vi "test Add Find Remove Analog Replay No VOverride.vi"(8 "error in (no error)":errorcluster, 11 "TestCase in":refnum<class "Scripting API Test Case.lvclass">) -> (0 "error out":errorcluster, 3 "TestCase out":refnum<class "Scripting API Test Case.lvclass">)   [LabVIEW 2019, in "Scripting API Test Case.lvclass"]
uses:
  Scripting API Test Case.lvclass
  <vilib>/addons/_JKI Toolkits/VI Tester/TestCase.llb/TestCase.lvclass
  <vilib>/NI/VeriStand Custom Device Testing Tools/VeriStandTestUtilities/VeriStandTestUtilities.lvlib
  Scripting API/Engine Simulation Toolkit Scripting API.lvlib
  Scripting API/Custom Device/Engine Simulation Toolkit Custom Device Settings.ctl
  <userlib>/_OpenG.lib/file/file.llb/Append Path to Root if Relative - Scalar__ogtk.vi
  Scripting API/Bitfile/Bitfile.ctl
  Scripting API/Analog Replay/Analog Replay Settings.ctl
  System Explorer/FPGA Mem Size.ctl
  System Explorer/Engine Simulation Toolkit System Explorer.lvlib
  System Explorer/Position Reference.ctl
  System Explorer/Data Replay Data Selection Method.ctl
  Scripting API/Analog Replay/Analog Replay Data Options.ctl
  C:/Program Files (x86)/National Instruments/LabVIEW 2019/vi.lib/addons/_JKI Toolkits/VI Tester/TestCase.llb/TestCase.lvclass
panel:
  in  "Save?":bool
  out "Output Filename":string
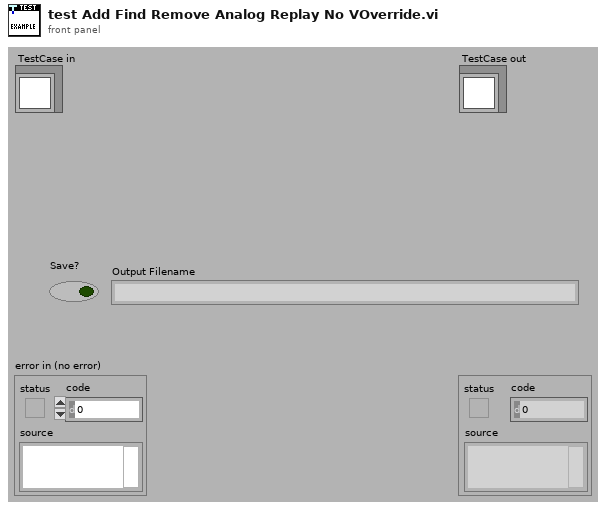
[diagram p1: front panel]
types:
  T1 = typedef "Engine Simulation Toolkit Scripting API.lvlib/Analog Replay Data Options.ctl" = cluster{"Selected File":path, "Group":string, "Channel":string, "DataPlugin":string, "ReverseData":bool, "FPGA memory size":T2, "CycleAngle?":T3, "Data Selection Method":T4, "File start offset":i32, "Samples":i32, "Missing teeth location (degrees)":dbl}
  T2 = typedef "Engine Simulation Toolkit System Explorer.lvlib/FPGA Mem Size.ctl" = enum16{"65,536", "32,768", "16,384", "8,192", "4,096", "2,048", "1,024"}
  T3 = typedef "Engine Simulation Toolkit System Explorer.lvlib/Position Reference.ctl" = enum16{"Crank angle", "Cycle angle"}
  T4 = typedef "Engine Simulation Toolkit System Explorer.lvlib/Data Replay Data Selection Method.ctl" = enum32{"Manual", "AutoVRCrank"}
  T5 = typedef "Engine Simulation Toolkit Scripting API.lvlib/Bitfile.ctl" = cluster{"RIO Device Address":string, "Bitfile Path":path}
  T6 = typedef "Engine Simulation Toolkit Scripting API.lvlib/Engine Simulation Toolkit Custom Device Settings.ctl" = cluster{"Name":string, "Execution priority":enum16{"Low", "Medium", "High"}, "Rate decimation":i32, "CPU":i32}
  T7 = typedef "Engine Simulation Toolkit Scripting API.lvlib/Analog Replay Settings.ctl" = cluster{"Name":string, "RIO Device Address":string, "DAC bipolar range (V)":dbl, "Voltage below min speed":dbl, "Min speed (RPM)":dbl, "Voltage at min speed":dbl, "Max speed (RPM)":dbl, "Voltage at max speed":dbl, "ReverseNegate":bool, "VOverride":bool}
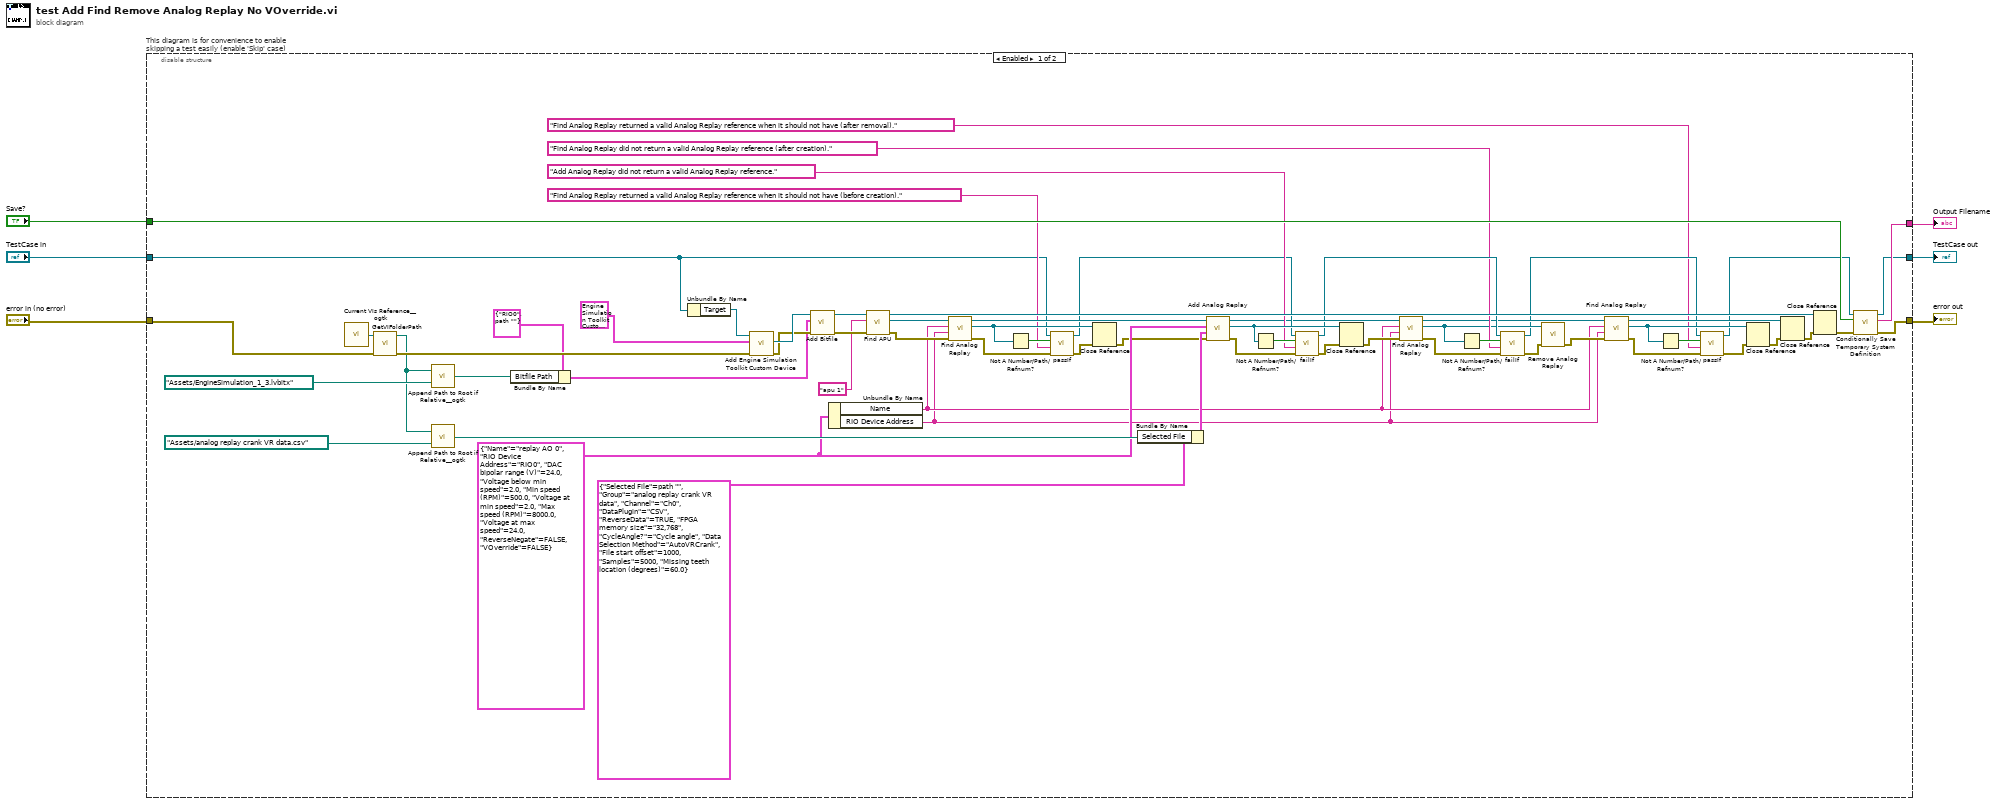
[diagram p0: block diagram]
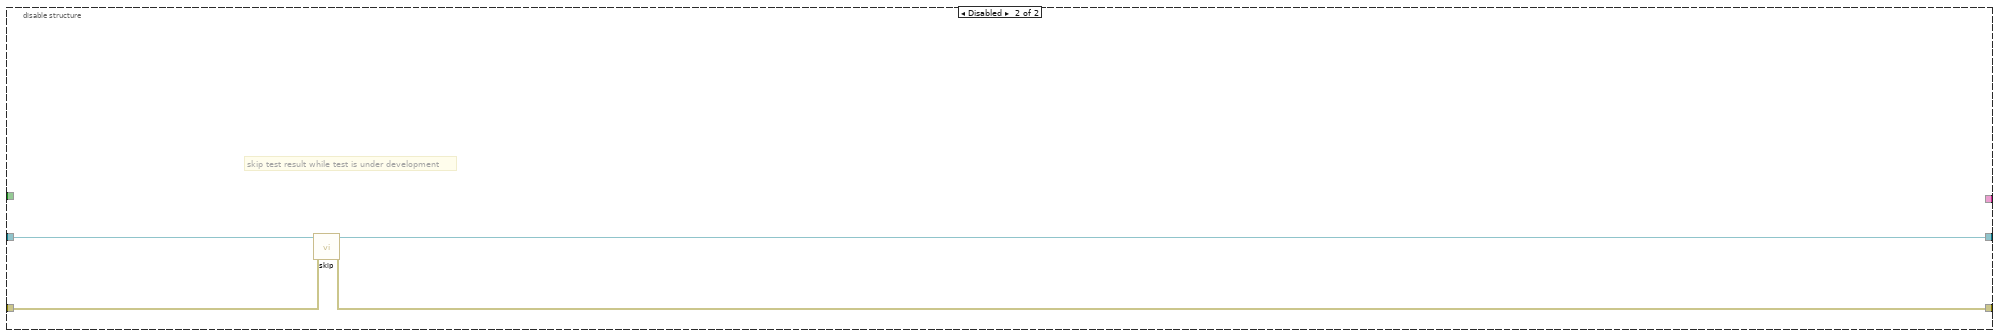
[diagram p2: hidden frame]
diagram:
  n1 = disable-structure "This diagram is for convenience to enable skipping a test easily (enable 'Skip' case)" shown="Enabled" {
    disable-tunnel: "TestCase in" -> [w8 w74]
    disable-tunnel: [w9 w72] -> w3
    disable-tunnel: [w66 w73] -> w5
    disable-tunnel: "error in (no error)" -> [w69 w71]
    disable-tunnel: [w65 _] -> w2
    disable-tunnel: "Save?" -> [w64 _]
    frame Enabled {
      w41 = T7 {"Name"="replay AO 0", "RIO Device Address"="RIO0", "DAC bipolar range (V)"=24.0, "Voltage below min speed"=2.0, "Min speed (RPM)"=500.0, "Voltage at min speed"=2.0, "Max speed (RPM)"=8000.0, "Voltage at max speed"=24.0, "ReverseNegate"=FALSE, "VOverride"=FALSE} ("Analog Replay Settings")
      n2 = call <userlib>:"Current VIs Reference__ogtk.vi"() -> ("Current VI's reference"=w70:refnum<vi>)  [unwired: 5 in]
      n3 = call <vilib>:"GetVIFolderPath.vi"("error in (no error)"=w69, "VI Reference in"=w70) -> ("error out"=w68:errorcluster, "VI Folder Path out"=w49:path)  [unwired: 8 in]
      n4 = call-poly <userlib>:"Append Path to Root if Relative__ogtk.vi"("Absolute or Relative Path"=path "Assets/EngineSimulation_1_3.lvbitx", "Root Path"=w49) -> ("Absolute or Appended Path"=w57:path)
      n5 = call-poly <userlib>:"Append Path to Root if Relative__ogtk.vi"("Absolute or Relative Path"=path "Assets/analog replay crank VR data.csv", "Root Path"=w49) -> ("Absolute or Appended Path"=w48:path)
      n6 = Bundle By Name(cluster=T5 {"RIO Device Address"="RIO0", "Bitfile Path"=path ""} ("Engine Simulation Toolkit Bitfile"), "Bitfile Path"=w57) -> (w58:T5)
      n7 = Unbundle By Name(w8) -> ("Target"=w7:refnum<k24>)
      n8 = call "Add Engine Simulation Toolkit Custom Device.vi"("error in (no error)"=w68, "Settings"=T6 {"Name"="Engine Simulation Toolkit Custom Device", "Execution priority"=enum."Medium", "Rate decimation"=1, "CPU"=-2} ("Engine Simulation Toolkit Custom Device Settings"), "Target in"=w7) -> ("error out"=w61:errorcluster, "EST Custom Device"=w63:refnum<k24>)  [unwired: 6 in, 1 out]
      n9 = call "Add Bitfile.vi"("error in (no error)"=w61, "Engine Simulation Toolkit Bitfile"=w58, "EST Custom Device in"=w63) -> ("error out"=w55:errorcluster, "EST Custom Device out"=w56:refnum<k24>)  [unwired: 7 in]
      n10 = Unbundle By Name(w41) -> ("Name"=w20:string, "RIO Device Address"=w19:string)
      n11 = call "Find APU.vi"("error in (no error)"=w55, "Name"="apu 1", "EST Custom Device in"=w56) -> ("error out"=w38:errorcluster, "APU"=w40:refnum<k24>, "EST Custom Device out"=w54:refnum<k24>)  [unwired: 6 in]
      n12 = call "Find Analog Replay.vi"("error in (no error)"=w38, "RIO Device Address"=w19, "Name"=w20, "APU in"=w40) -> ("error out"=w34:errorcluster, "Analog Replay"=w36:refnum<k24>, "APU out"=w39:refnum<k24>)  [unwired: 5 in]
      n13 = Not A Number/Path/Refnum?(number/path/refnum=w36) -> (NaN/Path/Refnum?=w37:bool)
      n14 = call-dynamic "passIf.vi"("error in (no error)"=w34, "message (\"\")"="Find Analog Replay returned a valid Analog Replay reference when it should not have (before creation)." ("message (\"\")"), "pass"=w37, "TestCase in"=w8) -> ("error out"=w35:errorcluster, "TestCase out"=w33:refnum<class "Scripting API Test Case.lvclass">)  [unwired: 6 in]
      n15 = Close Reference(reference=w36, error in (no error)=w35) -> (error out=w31:errorcluster)
      n16 = Bundle By Name(cluster=T1 {"Selected File"=path "", "Group"="analog replay crank VR data", "Channel"="Ch0", "DataPlugin"="CSV", "ReverseData"=TRUE, "FPGA memory size"=enum."32,768", "CycleAngle?"=enum."Cycle angle", "Data Selection Method"=enum."AutoVRCrank", "File start offset"=1000, "Samples"=5000, "Missing teeth location (degrees)"=60.0} ("Analog Replay Data Options"), "Selected File"=w48) -> (w50:T1)
      n17 = call "Add Analog Replay.vi"("error in (no error)"=w31, "Analog Replay Data Options"=w50, "Analog Replay Settings"=w41, "APU in"=w39) -> ("error out"=w45:errorcluster, "Analog Replay"=w44:refnum<k24>, "APU out"=w28:refnum<k24>)  [unwired: 5 in]
      n18 = Not A Number/Path/Refnum?(number/path/refnum=w44) -> (NaN/Path/Refnum?=w46:bool)
      n19 = call-dynamic "failIf.vi"("error in (no error)"=w45, "message (\"\")"="Add Analog Replay did not return a valid Analog Replay reference." ("message (\"\")"), "fail"=w46, "TestCase in"=w33) -> ("error out"=w42:errorcluster, "TestCase out"=w26:refnum<class "Scripting API Test Case.lvclass">)  [unwired: 6 in]
      n20 = Close Reference(reference=w44, error in (no error)=w42) -> (error out=w27:errorcluster)
      n21 = call "Find Analog Replay.vi"("error in (no error)"=w27, "RIO Device Address"=w19, "Name"=w20, "APU in"=w28) -> ("error out"=w29:errorcluster, "Analog Replay"=w24:refnum<k24>, "APU out"=w22:refnum<k24>)  [unwired: 5 in]
      n22 = Not A Number/Path/Refnum?(number/path/refnum=w24) -> (NaN/Path/Refnum?=w30:bool)
      n23 = call-dynamic "failIf.vi"("error in (no error)"=w29, "message (\"\")"="Find Analog Replay did not return a valid Analog Replay reference (after creation)." ("message (\"\")"), "fail"=w30, "TestCase in"=w26) -> ("error out"=w23:errorcluster, "TestCase out"=w13:refnum<class "Scripting API Test Case.lvclass">)  [unwired: 6 in]
      n24 = call "Remove Analog Replay.vi"("error in (no error)"=w23, "Analog Replay"=w24) -> ("error out"=w21:errorcluster)  [unwired: 9 in]
      n25 = call "Find Analog Replay.vi"("error in (no error)"=w21, "RIO Device Address"=w19, "Name"=w20, "APU in"=w22) -> ("error out"=w11:errorcluster, "Analog Replay"=w17:refnum<k24>, "APU out"=w15:refnum<k24>)  [unwired: 5 in]
      n26 = Not A Number/Path/Refnum?(number/path/refnum=w17) -> (NaN/Path/Refnum?=w18:bool)
      n27 = call-dynamic "passIf.vi"("error in (no error)"=w11, "message (\"\")"="Find Analog Replay returned a valid Analog Replay reference when it should not have (after removal)." ("message (\"\")"), "pass"=w18, "TestCase in"=w13) -> ("error out"=w16:errorcluster, "TestCase out"=w10:refnum<class "Scripting API Test Case.lvclass">)  [unwired: 6 in]
      n28 = Close Reference(reference=w17, error in (no error)=w16) -> (error out=w14:errorcluster)
      n29 = Close Reference(reference=w15, error in (no error)=w14) -> (error out=w52:errorcluster)
      n30 = Close Reference(reference=w54, error in (no error)=w52) -> (error out=w67:errorcluster)
      n31 = call "Conditionally Save Temporary System Definition.vi"("error in (no error)"=w67, "Save?"=w64, "Test Case"=w10) -> ("error out"=w66:errorcluster, "filename"=w65:string, "Test Case"=w9:refnum<class "Scripting API Test Case.lvclass">)  [unwired: 6 in]
    }
    frame Disabled {
      # "skip test result while test is under development"
      n32 = call <vilib>:"skip.vi"("error in (no error)"=w71, "TestCase in"=w74) -> ("error out"=w73:errorcluster, "TestCase out"=w72:refnum<class "Scripting API Test Case.lvclass">)  [unwired: 8 in]
    }
  }
  "error out" <- w5
  "TestCase out" <- w3
  "Output Filename" <- w2
